vi "LVClass_HasoEngine Get Spots Positions.vi"(0 "HasoEngine in":refnum<class "HasoEngine.lvclass">, 11 "error in (no error)":errorcluster) -> (4 "HasoEngine out":refnum<class "HasoEngine.lvclass">, 6 "pixX":i32, 10 "pixY":i32, 15 "error out":errorcluster)   [LabVIEW 2020, in "HasoEngine.lvclass"]
doc: "int32_t Imop_HasoEngine_GetSpotsPositions(CStr message, int32_t objet, int32_t pixX, int32_t pixY);"
uses:
  HasoEngine.lvclass
  HasoEngine.lvclass/HasoEngine.ctl
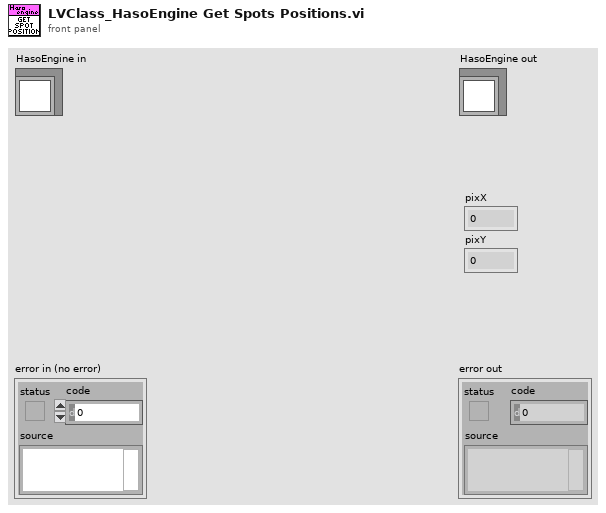
[diagram p1: front panel]
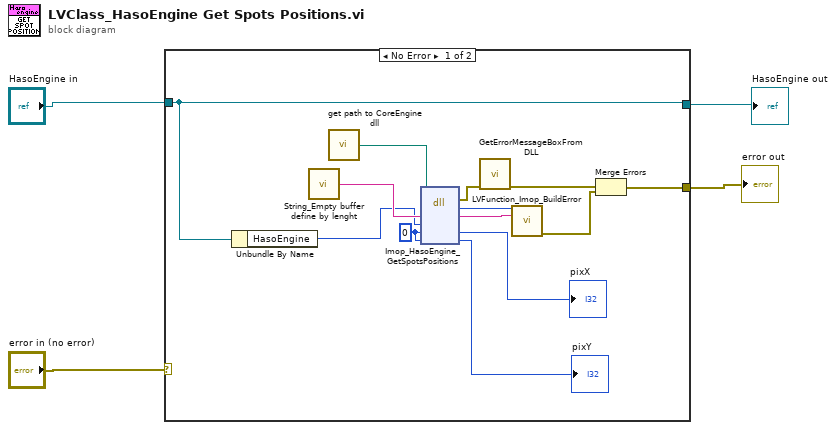
[diagram p0: block diagram]
diagram:
  n1 = case shown="No Error" "error in (no error)" {
    selector: "error in (no error)" -> [_ w18]
    tunnel: "HasoEngine in" -> [w9 w19]
    tunnel: [w9 w19] -> w1
    tunnel: [w5 w18] -> w2
    frame No Error {
      w14 = 0 ("pixX")
      n2 = Unbundle By Name(w9) -> ("HasoEngine"=w8:i32)
      n3 = call "String_Empty buffer define by lenght.vi"() -> ("Empty buffer"=w17:string)  [unwired: 1 in]
      n4 = call "get path to CoreEngine dll.vi"() -> ("path to c_interface_vc100.dll"=w11:path)  [unwired: 12 in, 3 out]
      n5 = dll-call lib="D:/2_trunk/Soft_haso/ImOpCoreEngine4_LV2011/DLLs/ImopEngine4_vc100.dll" fn="Imop_HasoEngine_GetSpotsPositions"(path in=w11, "message"=w17, "objet"=w8, "pixX"=w14, "pixY"=w14) -> (error out=w10:errorcluster, "return type"=w15:i32, "message"=w16:string, "pixX"=→"pixX":i32, "pixY"=→"pixY":i32)  [unwired: 3 in, 1 out]
      n6 = call "GetErrorMessageBoxFromDLL.vi"("error IN"=w10) -> ("error OUT"=w7:errorcluster)  [unwired: 10 in]
      n7 = call "LVFunction_Imop_BuildError.vi"("code"=w15, "String to Prepend to source (\"\")"=w16) -> ("error out"=w6:errorcluster)  [unwired: 13 in]
      n8 = Merge Errors(w7, w6) -> (w5:errorcluster)
    }
    frame Error {
    }
  }
  "error out" <- w2
  "HasoEngine out" <- w1
